vi "UHR-Fleezers Control (host) - Lorentz v5.vi"() -> ()   [LabVIEW 2014] (continued)
                  frame Enabled {
                  }
                }
                n2227 = local read "Actual MCL Inc (V)"() -> (w3371:dbl)
                n2228 = local read "Scan steps (MCL)"() -> (w3376:u64)
                n2229 = Divide "Y Pix/step"(x=w3372, y=w3377) -> (x/y=w3384:dbl)
                n2230 = Divide "Y V/pix"(x=w3371, y=w3384) -> (x/y=w3383:dbl)
                n2231 = Divide "Y half step offset"(x=w3371, y=2.0) -> (x/y=w3385:dbl)
                n2232 = Divide "X pix/step"(x=w3373, y=w3376) -> (x/y=w3382:dbl)
                n2233 = Negate(x=w3385) -> (-x=w3386:dbl)
                n2234 = local read "Initial Y"() -> (w3392:dbl)
                n2235 = Multiply(x=w3374, y=w3383) -> (x*y=w3393:dbl)
                n2236 = Divide "X half step offset"(x=w3371, y=2.0) -> (x/y=w3379:dbl)
                n2237 = Divide "X V/pix"(x=w3371, y=w3382) -> (x/y=w3381:dbl)
                n2238 = Multiply(x=w3371, y=w3376) -> (x*y=w3388:dbl)
                n2239 = Compound Arithmetic op=ADD(w3386, w3393, w3392) -> (w3363:dbl)
                "Pointer Y (V)" <- w3363
                n2240 = Multiply(x=w3381, y=w3375) -> (x*y=w3390:dbl)
                n2241 = Negate(x=w3379) -> (-x=w3378:dbl)
                n2242 = local read "Initial X"() -> (w3391:dbl)
                n2243 = Negate(x=w3390) -> (-x=w3389:dbl)
                n2244 = Compound Arithmetic op=ADD(w3378, w3388, w3391, w3389) -> (w3364:dbl)
                "Pointer X (V)" <- w3364
                n2245 = case shown="True" "Set High F Confocal Spot (X-Y)" {
                  tunnel: w3364 -> [_ w3394]
                  tunnel: w3363 -> [_ w3395]
                  frame False {
                  }
                  frame True {
                    "Confocal Y 2 (V)" <- w3395
                    "Confocal X 2 (V)" <- w3394
                  }
                }
                n2246 = Or(x="Set X Only", y="Set Confocal Spot (X-Y)") -> (x .or. y?=w3367:bool)
                n2247 = Or(x="Set Confocal Spot (X-Y)", y="Set Y Only") -> (x .or. y?=w3366:bool)
                n2248 = case shown="True" w3367 {
                  tunnel: w3364 -> [_ w3396]
                  frame False {
                  }
                  frame True {
                    n2249 = property on="AO2" class="Slide (strict)"("Val(Sgnl)"=w3396) -> ()  [unwired: 2 in, 2 out]
                    "Confocal X 1 (V)" <- w3396
                  }
                }
                n2250 = case shown="True" w3366 {
                  tunnel: w3363 -> [_ w3397]
                  frame False {
                  }
                  frame True {
                    n2251 = property on="AO1" class="Slide (strict)"("Val(Sgnl)"=w3397) -> ()  [unwired: 2 in, 2 out]
                    "Confocal Y 1 (V)" <- w3397
                  }
                }
                n2252 = local write "Set High F Confocal Spot (X-Y)"(w3362) -> ()
                n2253 = local write "Set Confocal Spot (X-Y)"(w3362) -> ()
                n2254 = local write "Set X Only"(w3362) -> ()
                n2255 = local write "Set Y Only"(w3362) -> ()
              }
            }
          }
          frame 3 {
            n2256 = local read "BD 2 Frequency 1 (MHz)"() -> (w3399:dbl)
            n2257 = local read "BD 1 Frequency 1 (MHz)"() -> (w3400:dbl)
            n2258 = local write "Manipulating Trap"(TRUE ("Manipulating Trap")) -> ()
            n2259 = local write "Coords"(T12 {"Horizontal"=0, "Vertical"=0} ("Coords")) -> ()
            n2260 = while {
              tunnel: w3404 -> [w3409]
              tunnel: w3402 -> [w3408]
              tunnel: w3400 -> [w3407]
              tunnel: w3399 -> [w3406]
              tunnel: w3398 -> [w3405]
              stop <- w3410 stop-if-true
              n2261 = event shown="[0] \"Pane\": Mouse Move" {
                selector: _ -> [_ _]
                dyn-events: _ -> [_ _]
                timeout: _ -> [_ _]
                tunnel: ["Force Manip Abort" w3474] -> w3410
                tunnel: w3409 -> [w3417 _]
                tunnel: w3408 -> [w3415 _]
                tunnel: w3407 -> [w3414 _]
                tunnel: w3406 -> [w3413 _]
                tunnel: w3405 -> [w3411 _]
                event Mouse Move {
                  n2262 = event-data() -> ("Time"=w3418:u32, "Coords"=w3419:T12)  [unwired: 3 out]
                  n2263 = Less?(x=w3418, y=w3417) -> (x < y?=w3416:bool)
                  n2264 = case "Makes sure old motion events prior to mouse click aren't used" shown="False" w3416 {
                    tunnel: w3419 -> [w3461 _]
                    tunnel: w3415 -> [w3462 _]
                    tunnel: w3414 -> [w3436 _]
                    tunnel: w3413 -> [w3435 _]
                    tunnel: w3411 -> [w3420 _]
                    frame False {
                      n2265 = Subtract(x=w3461, y=w3462) -> (x-y=w3460:T12)
                      "Coords" <- w3460
                      n2266 = local read "Y RF Frequency Limits (MHz)"() -> (w3421:T23)
                      n2267 = To Double Precision Float(number=w3460) -> (double precision float=w3459:cluster{"Horizontal":dbl, "Vertical":dbl})
                      n2268 = Multiply(x=cluster{"Horizontal":dbl, "Vertical":dbl} {"Horizontal"=-1.0, "Vertical"=1.0}, y="Manipulation Scaling") -> (x*y=w3455:cluster{"Horizontal":dbl, "Vertical":dbl})
                      n2269 = local read "X RF Frequency Limits (MHz)"() -> (w3422:T23)
                      n2270 = Multiply(x=w3459, y=w3455) -> (x*y=w3457:cluster{"Horizontal":dbl, "Vertical":dbl})
                      n2271 = Unbundle By Name(w3457) -> ("Horizontal"=w3452:dbl, "Vertical"=w3456:dbl)
                      n2272 = Unbundle By Name(w3421) -> ("Maximum"=w3424:dbl, "Minimum"=w3423:dbl)
                      n2273 = Boolean To (0,1)(Boolean="Manip. X?") -> (0, 1=w3450:i16)
                      n2274 = Boolean To (0,1)(Boolean="Manip. Y?") -> (0, 1=w3447:i16)
                      n2275 = local read "BD 1 Frequency 2 (MHz)"() -> (w3438:dbl)
                      n2276 = Multiply(x=w3456, y=w3447) -> (x*y=w3449:dbl)
                      n2277 = Multiply(x=w3450, y=w3452) -> (x*y=w3453:dbl)
                      n2278 = local read "BD 2 Frequency 2 (MHz)"() -> (w3437:dbl)
                      n2279 = Unbundle By Name(w3422) -> ("Maximum"=w3426:dbl, "Minimum"=w3425:dbl)
                      n2280 = Add(x=w3435, y=w3449) -> (x+y=w3428:dbl)
                      n2281 = Add(x=w3436, y=w3453) -> (x+y=w3430:dbl)
                      n2282 = In Range and Coerce(upper limit=w3426, x=w3430, lower limit=w3425) -> (coerced(x)=w3429:dbl)  [unwired: 1 out]
                      n2283 = In Range and Coerce(upper limit=w3424, x=w3428, lower limit=w3423) -> (coerced(x)=w3427:dbl)  [unwired: 1 out]
                      n2284 = Subtract(x=w3429, y=w3438) -> (x-y=w3446:dbl)
                      n2285 = Subtract(x=w3427, y=w3437) -> (x-y=w3445:dbl)
                      n2286 = Square(x=w3446) -> (x^2=w3444:dbl)
                      n2287 = Square(x=w3445) -> (x^2=w3443:dbl)
                      n2288 = Add(x=w3444, y=w3443) -> (x+y=w3442:dbl)
                      n2289 = Square Root(x=w3442) -> (sqrt(x)=w3439:dbl)
                      n2290 = In Range and Coerce(upper limit="Limit Max (MHz)", x=w3439, lower limit="Limit Min (MHz)") -> (In Range?=w3432:bool)  [unwired: 1 out]
                      n2291 = Not(x="Limits Enable") -> (.not. x?=w3431:bool)
                      n2292 = Or(x=w3432, y=w3431) -> (x .or. y?=w3433:bool)
                      n2293 = case shown="True" w3433 {
                        tunnel: w3439 -> [_ w3464]
                        tunnel: w3429 -> [_ w3471]
                        tunnel: w3438 -> [_ w3470]
                        tunnel: w3427 -> [_ w3469]
                        tunnel: w3437 -> [_ w3468]
                        tunnel: w3422 -> [_ w3466]
                        tunnel: w3421 -> [_ w3465]
                        tunnel: w3420 -> [_ w3463]
                        frame False {
                        }
                        frame True {
                          n2294 = local read "BD 1 Frequency 3 (MHz)"() -> (w3472:dbl)
                          n2295 = local read "BD 2 Frequency 3 (MHz)"() -> (w3467:dbl)
                          n2296 = local write "Trap Delta (MHz)"(w3464) -> ()
                          n2297 = call "set RF board frequency - interlace.vi"("Board 2 Frequency Limits"=w3465, "Board 1 Frequency Limits"=w3466, "FPGA VI Reference In"=w3463, "Board 2 Frequency 3 (MHz)"=w3467, "Board 1 Frequency 3 (MHz)"=w3472, "Board 2 Frequency 2 (MHz)"=w3468, "Board 2 Frequency 1 (MHz)"=w3469, "Board 1 Frequency 2 (MHz)"=w3470, "Board 1 Frequency 1  (MHz)"=w3471) -> ()  [unwired: 1 in, 2 out]
                          n2298 = local write "BD 2 Frequency 1 (MHz)"(w3469) -> ()
                          n2299 = local write "BD 1 Frequency 1 (MHz)"(w3471) -> ()
                        }
                      }
                    }
                    frame True {
                    }
                  }
                }
                event Mouse Up {
                  n2300 = event-data() -> ("Button"=w3473:u16)  [unwired: 8 out]
                  n2301 = case shown="3" w3473 {
                    tunnel: [FALSE TRUE] -> w3474
                    frame 0, Default {
                    }
                    frame 3 {
                      n2302 = local read "Trap Delta (MHz)"() -> (w3476:dbl)
                      n2303 = property on="Initial delta (MHz)" class="DigNum (strict)"("Val(Sgnl)"=w3476) -> ()  [unwired: 2 in, 2 out]
                      n2304 = local write "Manipulating Trap"(FALSE ("Manipulating Trap")) -> ()
                    }
                  }
                }
              }
            }
          }
        }
      }
      event Timeout {
        n2305 = event-data() -> ()  [unwired: 4 out]
      }
      event "Stop All": Mouse Down {
        n2306 = event-data() -> ()  [unwired: 9 out]
      }
      event Mouse Move {
        n2307 = event-data() -> ()  [unwired: 6 out]
      }
    }
    n2308 = node-c288() -> ()  [unwired: 2 out]
  }
  n2309 = node-c288(3 ("Processor")) -> (w60:T36)  [unwired: 3 out]
  n2310 = node-c288(i64 1 ("Period"), 1 ("Processor")) -> (w68:T36)  [unwired: 2 in, 2 out]
  n2311 = timed-loop "Oscillate Trap/AOM (fishing, conjugate plane alignment)" {
    tunnel: [w3482] -> w65
    timing: w60 -> [_]
    timing-out: [_] -> w59
    tunnel: w21 -> [w3481]
    tunnel: w9 -> [w3480]
    stop <- w3482 stop-if-true
    n2312 = node-c288() -> ()  [unwired: 2 out]
    n2313 = event shown="[2] \"Start assembly line\": Value Change" {
      selector: _ -> [_ _ _ _]
      dyn-events: _ -> [_ _ _ _]
      timeout: _ -> [_ _ _ _]
      tunnel: [FALSE ("Stop All") _ _ w4155] -> w3482
      tunnel: w3481 -> [w3485 _ _ _]
      tunnel: w3480 -> [_ _ w4090 _]
      event "Oscillate Set 1", "Fish for Tether": Value Change {
        n2314 = event-data() -> ()  [unwired: 6 out]
        n2315 = local read "Oscillate Set 1"() -> (w3489:bool)
        n2316 = Or(x=w3489, y="Fish for Tether") -> (x .or. y?=w3487:bool)
        n2317 = case shown="True" w3487 {
          tunnel: "Fish for Tether" -> [_ w3492]
          tunnel: w3485 -> [_ w3490]
          frame False {
          }
          frame True {
            n2318 = case shown="True" w3492 {
              selector: w3492 -> [w3495 w3501]
              tunnel: [w3495 w3501] -> w3491
              frame False {
              }
              frame True {
                n2319 = local write "Scan axis 2"(TRUE) -> ()
                n2320 = local write "Tether"(FALSE ("Tether")) -> ()
                n2321 = local read "Flow ON during cal?"() -> (w3496:bool)
                n2322 = property on="Trap Delta (MHz)" class="DigNum (strict)"("Val(Sgnl)"="Furthest Delta (MHz)") -> ()  [unwired: 2 in, 2 out]
                n2323 = Or(x="Flow ON during \nfishing?", y=w3496) -> (x .or. y?=w3497:bool)
                n2324 = Wait (ms)(milliseconds to wait=u32 500) -> ()  [unwired: 1 out]
                n2325 = property on="Sample Channel\nFlow" class="Bool (strict)"("Val(Sgnl)"=w3497) -> ()  [unwired: 2 in, 2 out]
              }
            }
            n2326 = node-c288() -> (w3494:T36)  [unwired: 1 in, 3 out]
            n2327 = timed-loop "Oscillate AOD" {
              timing: w3494 -> [_]
              timing-out: [_] -> w3493
              tunnel: w3491 -> [w3505]
              tunnel: w3490 -> [w3504]
              i -> [w3513]
              stop <- w3511 stop-if-true
              n2328 = node-c288() -> (w3512:i64)  [unwired: 1 out]
              n2329 = flat-sequence {
                tunnel: w3513 -> [w3540]
                tunnel: w3512 -> [w3539]
                tunnel: w3505 -> [w3523]
                tunnel: [w3523] -> w3510
                tunnel: [w3522] -> w3509
                tunnel: [w3521] -> w3508
                tunnel: [w3518] -> w3506
                tunnel: w3504 -> [w3514]
                tunnel: w3510 -> [w3587]
                tunnel: w3509 -> [w3585]
                tunnel: w3508 -> [w3584]
                tunnel: [w3583] -> w3507
                tunnel: w3506 -> [w3582]
                tunnel: [w3659] -> w3511
                tunnel: w3507 -> [w3658]
                frame #0 {
                  # "w (rad/s)"
                  # "t (s)"
                  n2330 = Divide(x=w3539, y=i64 1000) -> (x/y=w3515:dbl)
                  n2331 = local read "BD 1 Frequency 2 (MHz)"() -> (w3517:dbl)
                  n2332 = Multiply(x="Osc. freq. (Hz)", y=6.283185307179586) -> (x*y=w3537:dbl)
                  n2333 = Multiply(x=w3515, y=w3540) -> (x*y=w3536:dbl)
                  n2334 = Multiply(x=w3537, y=w3536) -> (x*y=w3520:dbl)
                  n2335 = local read "BD 1 Frequency 1 (MHz)"() -> (w3525:dbl)
                  n2336 = case shown="True" w3523 {
                    tunnel: w3520 -> [w3546 w3565]
                    tunnel: w3525 -> [_ w3573]
                    tunnel: w3517 -> [_ w3574]
                    tunnel: [w3543 w3569] -> w3516
                    tunnel: [FALSE w3547] -> w3521
                    tunnel: [0.0 w3561] -> w3518
                    frame False {
                      n2337 = Sine(x=w3546) -> (sin(x)=w3544:dbl)
                      n2338 = Multiply(x=w3544, y="Osc. amp. (MHz)") -> (x*y=w3543:dbl)
                    }
                    frame True {
                      # "trap position goes from 0 to 1 (0 is when it is furthest away, 1 is when closest)\nso we want to test for tether only when farther away, or x < 1"
                      # "quit if taking too long"
                      # "oscillate the trap"
                      # "Test for tether"
                      n2339 = local read "Vec Mean of T1 T2"() -> (w3550:dbl[])
                      "Trigger Signal" <- w3550
                      n2340 = Cosine(x=w3565) -> (cos(x)=w3577:dbl)
                      n2341 = Subtract(x=w3574, y=w3573) -> (x-y=w3572:dbl)
                      n2342 = Decrement(x=w3577) -> (x-1=w3576:dbl)
                      n2343 = Subtract(x=w3572, y="Closest Delta (MHz)") -> (x-y=w3570:dbl)
                      n2344 = Divide(x=w3576, y=-2.0) -> (x/y=w3560:dbl)
                      n2345 = Greater?(x=w3550, y="Stop F (pN)") -> (0:w3567:bool[])
                      n2346 = Multiply(x=w3560, y=w3570) -> (x*y=w3569:dbl)
                      n2347 = Less?(x=w3560, y="Fish mask thresh") -> (x < y?=w3559:bool)
                      n2348 = Boolean To (0,1)(Boolean=w3559) -> (0, 1=w3557:i16)
                      n2349 = Multiply(x=w3557, y=w3550) -> (x*y=w3556:dbl[])
                      n2350 = Divide(x=w3565, y=6.283185307179586) -> (x/y=w3564:dbl)
                      n2351 = Round Toward +Infinity(x=w3564) -> (ceil(x): smallest int >= x=w3561:dbl)
                      "Attempts" <- w3561
                      n2352 = Greater?(x=w3556, y="Stop F (pN) (mask)") -> (0:w3554:bool[])
                      n2353 = Or Array Elements(Boolean array=w3567) -> (logical OR=w3552:bool)
                      n2354 = Or Array Elements(Boolean array=w3554) -> (logical OR=w3551:bool)
                      n2355 = Greater?(x=w3561, y="Attempt Limit") -> (0:w3563:bool)
                      n2356 = case shown="True" w3563 {
                        frame False {
                        }
                        frame True {
                          n2357 = local write "Fish for Tether"(FALSE ("Fish for Tether")) -> ()
                          n2358 = call <vilib>:"Beep.vi"() -> ()  [unwired: 3 in, 9 out]
                          n2359 = local read "Messages"() -> (w3579:string)
                          n2360 = call "Update messages.vi"("Message to add"="Tether fishing timeout." ("Messages"), "Old message string"=w3579) -> ("New message string"=→"Messages":string)
                        }
                      }
                      n2361 = Select(t=w3552, s="Normal (on) or masked test (off)", f=w3551) -> (s? t:f=w3549:bool)
                      n2362 = And(x="Stop Fishing When Tether", y=w3549) -> (x .and. y?=w3547:bool)
                    }
                  }
                  n2363 = local read "BD 2 Frequency 1 (MHz)"() -> (w3524:dbl)
                  n2364 = Select(t=w3525, s="Scan axis 2", f=w3524) -> (s? t:f=w3528:dbl)
                  n2365 = Add(x=w3516, y=w3528) -> (x+y=w3522:dbl)
                  n2366 = Select(t=w3522, s="Scan axis 2", f=w3525) -> (s? t:f=w3531:dbl)
                  n2367 = Select(t=w3524, s="Scan axis 2", f=w3522) -> (s? t:f=w3530:dbl)
                  n2368 = local read "BD 2 Frequency 2 (MHz)"() -> (w3533:dbl)
                  n2369 = local read "BD 2 Frequency 3 (MHz)"() -> (w3532:dbl)
                  n2370 = local read "Y RF Frequency Limits (MHz)"() -> (w3526:T23)
                  n2371 = local read "X RF Frequency Limits (MHz)"() -> (w3527:T23)
                  n2372 = local read "BD 1 Frequency 3 (MHz)"() -> (w3534:dbl)
                  n2373 = call "set RF board frequency - interlace.vi"("Board 2 Frequency Limits"=w3526, "Board 1 Frequency Limits"=w3527, "FPGA VI Reference In"=w3514, "Board 2 Frequency 3 (MHz)"=w3532, "Board 1 Frequency 3 (MHz)"=w3534, "Board 2 Frequency 2 (MHz)"=w3533, "Board 2 Frequency 1 (MHz)"=w3530, "Board 1 Frequency 2 (MHz)"=w3517, "Board 1 Frequency 1  (MHz)"=w3531) -> ()  [unwired: 1 in, 2 out]
                }
                frame #1 {
                  n2374 = And(x=w3587, y=w3584) -> (x .and. y?=w3586:bool)
                  n2375 = case "Only if were fishing and now formed tether" shown="True" w3586 {
                    tunnel: w3585 -> [w3589 w3604]
                    tunnel: [w3588 w3603] -> w3583
                    tunnel: w3582 -> [_ w3599]
                    frame False {
                      n2376 = local read "Fish for Tether"() -> (w3588:bool)
                      n2377 = case shown="False" w3588 {
                        tunnel: w3589 -> [w3590 _]
                        frame False {
                          n2378 = property on="BD 1 Frequency 1 (MHz)" class="DigNum (strict)"("Val(Sgnl)"=w3590) -> ()  [unwired: 2 in, 2 out]
                        }
                        frame True {
                        }
                      }
                    }
                    frame True {
                      w3603 = FALSE ("Fish for Tether")
                      n2379 = call <vilib>:"Beep.vi"() -> ()  [unwired: 3 in, 9 out]
                      n2380 = Number To Decimal String(number=w3599, width (-)=i16 1) -> (decimal integer string=w3597:string)
                      n2381 = Concatenate Strings("Formed tether in ", w3597, " attempt(s)." ("string")) -> (w3594:string)
                      n2382 = local read "Messages"() -> (w3601:string)
                      n2383 = local write "Fish for Tether"(w3603) -> ()
                      n2384 = call "Update messages.vi"("Message to add"=w3594, "Old message string"=w3601) -> ("New message string"=w3600:string)
                      n2385 = local write "Messages"(w3600) -> ()
                      n2386 = Get Date/Time In Seconds() -> (seconds since 1Jan1904=→"Time tether formed":timestamp)
                      n2387 = local read "Flow ON during cal?"() -> (w3591:bool)
                      n2388 = property on="Sample Channel\nFlow" class="Bool (strict)"("Val(Sgnl)"=w3591) -> (error out=w3592:errorcluster)  [unwired: 2 in, 1 out]
                      n2389 = case shown="\"2\", \"3\", \"4\", \"5\", \"6\"" "Then..." {
                        selector: "Then..." -> [_ w3607]
                        tunnel: w3604 -> [w3606 _]
                        tunnel: w3592 -> [_ _]
                        frame "1", Default {
                          n2390 = property on="BD 1 Frequency 1 (MHz)" class="DigNum (strict)"("Val(Sgnl)"=w3606) -> ()  [unwired: 2 in, 2 out]
                        }
                        frame "2", "3", "4", "5", "6" {
                          n2391 = flat-sequence {
                            tunnel: w3607 -> [w3609]
                            frame #0 {
                              n2392 = property on="Trap Delta (MHz)" class="DigNum (strict)"("Val(Sgnl)"="Move to Delta 1 (MHz)") -> ()  [unwired: 2 in, 2 out]
                            }
                            frame #1 {
                              n2393 = case shown="\"5\", \"6\"" w3609 {
                                selector: w3609 -> [w3612 w3622 _]
                                frame "3", "4" {
                                n2394 = flat-sequence {
                                tunnel: w3612 -> [w3613]
                                tunnel: [w3613] -> w3610
                                tunnel: [w3615] -> w3611
                                tunnel: w3610 -> [w3615]
                                tunnel: w3611 -> [w3619]
                                frame #0 {
                                n2395 = property on="Green Laser ON" class="Bool (strict)"("Val(Sgnl)"=TRUE ("Value (Signaling)")) -> ()  [unwired: 2 in, 2 out]
                                }
                                frame #1 {
                                n2396 = Multiply(x="Wait Before Save (s)", y=u32 1000 ("x")) -> (x*y=w3617:u32)
                                n2397 = Wait (ms)(milliseconds to wait=w3617) -> ()  [unwired: 1 out]
                                }
                                frame #2 {
                                n2398 = property on="Start Saving" class="Bool (strict)"("Value"=TRUE ("Start Saving")) -> ()  [unwired: 2 in, 2 out]
                                n2399 = case shown="\"4\"" w3619 {
                                frame Default {
                                }
                                frame "4" {
                                n2400 = property on="Fl. Triggered..." class="Bool (strict)"("Val(Sgnl)"=TRUE ("Value (Signaling)")) -> ()  [unwired: 2 in, 2 out]
                                }
                                }
                                }
                                }
                                }
                                frame "5", "6" {
                                n2401 = stacked-sequence {
                                tunnel: w3622 -> [_ _ _ _ _ _ w3634]
                                frame #0 {
                                n2402 = Replace Array Subset(array=u32[] [0] ("Index Values"), new element="Raster Set Upon Tether", index=0) -> (w3623:u32[])
                                n2403 = property on="Saved AOD Raster Scan Parameter Sets" class="Arr (strict)"("Index Values"=w3623) -> ()  [unwired: 2 in, 2 out]
                                }
                                frame #1 {
                                n2404 = Wait (ms)(milliseconds to wait=u32 500) -> ()  [unwired: 1 out]
                                }
                                frame #2 {
                                n2405 = property on="Load parameters" class="Bool (strict)"("Val(Sgnl)"=TRUE ("Value (Signaling)")) -> ()  [unwired: 2 in, 2 out]
                                n2406 = case shown="True" "Green ON During Raster" {
                                frame False {
                                }
                                frame True {
                                n2407 = property on="Green Laser ON" class="Bool (strict)"("Val(Sgnl)"=TRUE ("Value (Signaling)")) -> ()  [unwired: 2 in, 2 out]
                                }
                                }
                                }
                                frame #3 {
                                n2408 = Wait (ms)(milliseconds to wait=u32 500) -> ()  [unwired: 1 out]
                                }
                                frame #4 {
                                n2409 = property on="Trap Raster Scan" class="Bool (strict)"("Val(Sgnl)"=TRUE ("Value (Signaling)")) -> ()  [unwired: 2 in, 2 out]
                                }
                                frame #5 {
                                n2410 = Wait (ms)(milliseconds to wait=u32 2000) -> ()  [unwired: 1 out]
                                }
                                frame #6 {
                                n2411 = flat-sequence {
                                tunnel: w3634 -> [w3641]
                                frame #0 {
                                n2412 = while {
                                stop <- w3637 stop-if-true
                                n2413 = local read "Raster Scanning..."() -> (w3636:bool)
                                n2414 = local read "Saving..."() -> (w3639:bool)
                                n2415 = Wait (ms)(milliseconds to wait=u32 100) -> ()  [unwired: 1 out]
                                n2416 = Not(x=w3639) -> (.not. x?=w3638:bool)
                                n2417 = Not(x=w3636) -> (.not. x?=w3635:bool)
                                n2418 = And(x=w3638, y=w3635) -> (x .and. y?=w3637:bool)
                                }
                                }
                                frame #1 {
                                n2419 = local read "Tether"() -> (w3642:bool)
                                n2420 = case shown="True" w3642 {
                                tunnel: w3641 -> [_ w3644]
                                frame False {
                                n2421 = property on="Fish for Tether" class="Bool (strict)"("Val(Sgnl)"="Fish again after \nraster break?") -> ()  [unwired: 2 in, 2 out]
                                }
                                frame True {
                                n2422 = stacked-sequence {
                                tunnel: w3644 -> [_ w3648 _ _]
                                frame #0 {
                                n2423 = property on="Trap Delta (MHz)" class="DigNum (strict)"("Val(Sgnl)"="Move to Delta 2 (MHz)") -> ()  [unwired: 2 in, 2 out]
                                n2424 = case shown="True" "Flow ON after\ntether testing?" {
                                frame False {
                                }
                                frame True {
                                n2425 = property on="Sample Channel\nFlow" class="Bool (strict)"("Val(Sgnl)"=TRUE ("Value (Signaling)")) -> ()  [unwired: 2 in, 2 out]
                                }
                                }
                                }
                                frame #1 {
                                n2426 = flat-sequence {
                                tunnel: w3648 -> [w3650]
                                frame #0 {
                                n2427 = Wait (ms)(milliseconds to wait=u32 500) -> ()  [unwired: 1 out]
                                }
                                frame #1 {
                                n2428 = case shown="\"6\"" w3650 {
                                frame Default {
                                }
                                frame "6" {
                                n2429 = property on="Green Laser ON" class="Bool (strict)"("Val(Sgnl)"=TRUE ("Green Laser ON/Interlacing")) -> ()  [unwired: 2 in, 2 out]
                                }
                                }
                                }
                                frame #2 {
                                n2430 = Wait (ms)(milliseconds to wait=u32 500) -> ()  [unwired: 1 out]
                                }
                                frame #3 {
                                n2431 = local write "Start Saving"("Save at end (5, 6)") -> ()
                                }
                                }
                                }
                                frame #2 {
                                n2432 = local read "Bead Sep. Int. Time (s)"() -> (w3656:dbl)
                                n2433 = Multiply(x=w3656, y=1000.0) -> (x*y=w3655:dbl)
                                n2434 = Wait (ms)(milliseconds to wait=w3655) -> ()  [unwired: 1 out]
                                }
                                frame #3 {
                                n2435 = property on="Remove Offset" class="Bool (strict)"("Val(Sgnl)"=TRUE ("Value (Signaling)")) -> ()  [unwired: 2 in, 2 out]
                                }
                                }
                                }
                                }
                                }
                                }
                                }
                                }
                                }
                                frame "2", Default {
                                }
                              }
                            }
                          }
                        }
                      }
                      "Tether" <- "Tether Alarm?"
                    }
                  }
                }
                frame #2 {
                  n2436 = local read "Oscillate Set 1"() -> (w3663:bool)
                  n2437 = local read "Stop All"() -> (w3661:bool)
                  n2438 = Or(x=w3663, y=w3658) -> (x .or. y?=w3660:bool)
                  n2439 = Not(x=w3660) -> (.not. x?=w3662:bool)
                  n2440 = Compound Arithmetic op=OR(w3661, w3662) -> (w3659:bool)
                }
              }
              n2441 = node-c288() -> ()  [unwired: 2 out]
            }
            n2442 = node-c288(w3493) -> ()  [unwired: 1 out]
          }
        }
      }
      event "Fl. Triggered...": Value Change {
        n2443 = event-data() -> ()  [unwired: 7 out]
        n2444 = case shown="True" "Fl. Triggered..." {
          frame False {
          }
          frame True {
            n2445 = node-c288() -> (w3674:T36)  [unwired: 4 out]
            n2446 = timed-loop {
              timing: w3674 -> [_]
              timing-out: [_] -> w3673
              tunnel: "Action" -> [w3682]
              shift-right: [w3679] -> _
              shift-left: u8 255 -> [w3681]
              shift-right: [w3676] -> _
              shift-left: 255 -> [w3678]
              stop <- w3675 stop-if-true
              # "Reset confocal spot"
              n2447 = node-c288() -> ()  [unwired: 2 out]
              n2448 = flat-sequence {
                tunnel: w3682 -> [w3702]
                tunnel: w3681 -> [w3701]
                tunnel: [w3700] -> w3680
                tunnel: w3678 -> [w3687]
                tunnel: [w3686] -> w3677
                tunnel: [w4081] -> w3675
                tunnel: w3680 -> [w4080]
                tunnel: [w4080] -> w3679
                tunnel: [w4079] -> w3676
                tunnel: w3677 -> [w4079]
                frame #0 {
                  n2449 = local read "Delta Fl. 2"() -> (w3699:dbl)
                  n2450 = local read "Delta Fl. 1"() -> (w3694:dbl)
                  n2451 = Multiply(x="Fl. Delta Thresh. (kHz)", y=1000.0) -> (x*y=w3689:dbl)
                  n2452 = Select(t=w3694, s="APD to Watch", f=w3699) -> (s? t:f=w3690:dbl)
                  n2453 = Greater?(x=w3690, y=w3689) -> (0:w3695:bool)
                  n2454 = Or(x="Force Yank", y=w3695) -> (x .or. y?=w3693:bool)
                  n2455 = And(x=w3693, y="Yank when?") -> (x .and. y?=w3691:bool)
                  n2456 = case shown="True" w3691 {
                    tunnel: w3702 -> [w3705 w3906]
                    tunnel: w3701 -> [w3707 w3902]
                    tunnel: [w3707 w3900] -> w3700
                    tunnel: w3690 -> [w3713 _]
                    tunnel: w3689 -> [w3712 _]
                    tunnel: "Force Yank" -> [w3710 _]
                    tunnel: w3687 -> [w3709 w3899]
                    tunnel: [w3708 w3899] -> w3686
                    frame False {
                      n2457 = Negate(x=w3712) -> (-x=w3704:dbl)
                      n2458 = local write "Fl. High"(TRUE ("Fl. High")) -> ()
                      n2459 = Less?(x=w3713, y=w3704) -> (x < y?=w3711:bool)
                      n2460 = Or(x=w3710, y=w3711) -> (x .or. y?=w3706:bool)
                      n2461 = case shown="True" w3706 {
                        tunnel: w3709 -> [w3714 w3724]
                        tunnel: [w3714 w3723] -> w3708
                        tunnel: w3705 -> [_ w3722]
                        frame False {
                        }
                        frame True {
                          n2462 = flat-sequence {
                            tunnel: w3724 -> [w3730]
                            tunnel: w3722 -> [w3727]
                            tunnel: [w3729] -> w3721
                            tunnel: [w3728] -> w3720
                            tunnel: [w3727] -> w3719
                            tunnel: w3718 -> [w3726]
                            tunnel: [w3726] -> w3717
                            tunnel: w3716 -> [w3725]
                            tunnel: [w3725] -> w3715
                            tunnel: [w3801] -> w3723
                            tunnel: w3721 -> [w3801]
                            tunnel: w3720 -> [w3800]
                            tunnel: w3719 -> [w3799]
                            tunnel: w3717 -> [w3798]
                            tunnel: w3715 -> [w3797]
                            frame #0 {
                              n2463 = call <vilib>:"Beep.vi"() -> ()  [unwired: 12 in]
                              n2464 = local write "Waiting"(FALSE ("Waiting")) -> ()
                              n2465 = Increment(x=w3730) -> (x+1=w3729:i32)
                              n2466 = case shown="\"Image\"" w3727 {
                                tunnel: w3729 -> [_ w3735 _]
                                frame "Alarm", Default {
                                }
                                frame "Yank" {
                                n2467 = flat-sequence {
                                tunnel: w3735 -> [w3738]
                                tunnel: [w3737] -> w3734
                                tunnel: [w3736] -> w3733
                                tunnel: w3734 -> [w3748]
                                tunnel: w3733 -> [w3749]
                                frame #0 {
                                n2468 = local read "Yank Delay (s)"() -> (w3741:dbl)
                                n2469 = local read "N Array El"() -> (w3736:u8)
                                n2470 = Quotient & Remainder(x=w3738, y=w3736) -> (x-y*floor(x/y)=w3737:i32)  [unwired: 1 out]
                                n2471 = Multiply(x=w3741, y=1000.0) -> (x*y=w3739:dbl)
                                n2472 = Wait (ms)(milliseconds to wait=w3739) -> ()  [unwired: 1 out]
                                }
                                frame #1 {
                                n2473 = local read "Yank to which?"() -> (w3743:bool)
                                n2474 = local read "Random Choice"() -> (w3753:bool)
                                n2475 = local read "Yank to Trap Delta (MHz)"() -> (w3746:dbl[])
                                n2476 = local read "Yank to SP"() -> (w3747:dbl[])
                                n2477 = Random Number (0-1)() -> (number: 0 to 1=w3752:dbl)
                                n2478 = Multiply(x=w3749, y=w3752) -> (x*y=w3751:dbl)
                                n2479 = Round Toward -Infinity(1:w3751) -> (0:w3750:dbl)
                                n2480 = Select(t=w3750, s=w3753, f=w3748) -> (s? t:f=w3744:dbl)
                                n2481 = Select(t=w3746, s=w3743, f=w3747) -> (s? t:f=w3745:dbl[])
                                n2482 = Index Array(array=w3745, index=w3744) -> (element=w3742:dbl)
                                n2483 = case shown="True" w3743 {
                                tunnel: w3742 -> [w3754 w3781]
                                frame False {
                                n2484 = flat-sequence {
                                tunnel: w3754 -> [w3755]
                                frame #0 {
                                n2485 = property on="Trap Pos FB SP" class="DigNum (strict)"("Val(Sgnl)"=w3755) -> ()  [unwired: 2 in, 2 out]
                                }
                                frame #1 {
                                n2486 = Wait (ms)(milliseconds to wait=u32 700) -> ()  [unwired: 1 out]
                                }
                                frame #2 {
                                n2487 = local read "Action (%)"() -> (w3760:dbl)
                                n2488 = Absolute Value(x=w3760) -> (abs(x)=w3759:dbl)
                                n2489 = Greater?(x=w3759, y=70.0) -> (0:w3757:bool)
                                n2490 = property on="Remove Action Offset" class="Bool (strict)"("Val(Sgnl)"=w3757) -> ()  [unwired: 2 in, 2 out]
                                }
                                frame #3 {
                                n2491 = for {
                                N: 4 -> [_]
                                n2492 = flat-sequence {
                                frame #0 {
                                n2493 = Wait (ms)(milliseconds to wait=u32 500) -> ()  [unwired: 1 out]
                                }
                                frame #1 {
                                n2494 = local read "Action (%)"() -> (w3766:dbl)
                                n2495 = Absolute Value(x=w3766) -> (abs(x)=w3765:dbl)
                                n2496 = Greater?(x=w3765, y=70.0) -> (0:w3763:bool)
                                n2497 = property on="Remove Action Offset" class="Bool (strict)"("Val(Sgnl)"=w3763) -> ()  [unwired: 2 in, 2 out]
                                }
                                }
                                }
                                }
                                frame #4 {
                                n2498 = Wait (ms)(milliseconds to wait=u32 500) -> ()  [unwired: 1 out]
                                }
                                frame #5 {
                                n2499 = local read "Mean"() -> (w3774:dbl)
                                n2500 = Greater?(x=w3774, y=11.0) -> (0:w3768:bool)
                                n2501 = Not(x=w3768) -> (.not. x?=w3769:bool)
                                n2502 = And(x=w3769, y="Shift confocal") -> (x .and. y?=w3771:bool)
                                n2503 = And(x=w3768, y="Shift confocal") -> (x .and. y?=w3772:bool)
                                n2504 = case shown="True" w3772 {
                                frame False {
                                }
                                frame True {
                                n2505 = local read "Confocal Y 2 (V)"() -> (w3778:dbl)
                                n2506 = local read "Confocal X 2 (V)"() -> (w3777:dbl)
                                n2507 = property on="AO1" class="Slide (strict)"("Val(Sgnl)"=w3778) -> ()  [unwired: 2 in, 2 out]
                                n2508 = property on="AO2" class="Slide (strict)"("Val(Sgnl)"=w3777) -> ()  [unwired: 2 in, 2 out]
                                }
                                }
                                n2509 = case shown="True" w3771 {
                                frame False {
                                }
                                frame True {
                                n2510 = local read "Confocal Y 1 (V)"() -> (w3776:dbl)
                                n2511 = local read "Confocal X 1 (V)"() -> (w3775:dbl)
                                n2512 = property on="AO1" class="Slide (strict)"("Val(Sgnl)"=w3776) -> ()  [unwired: 2 in, 2 out]
                                n2513 = property on="AO2" class="Slide (strict)"("Val(Sgnl)"=w3775) -> ()  [unwired: 2 in, 2 out]
                                }
                                }
                                }
                                frame #6 {
                                n2514 = Wait (ms)(milliseconds to wait=u32 1500) -> ()  [unwired: 1 out]
                                }
                                frame #7 {
                                n2515 = property on="Rem fb disp offset" class="Bool (strict)"("Val(Sgnl)"=TRUE ("Value (Signaling)")) -> ()  [unwired: 2 in, 2 out]
                                }
                                }
                                }
                                frame True {
                                n2516 = flat-sequence {
                                tunnel: w3781 -> [w3782]
                                frame #0 {
                                n2517 = property on="Trap Delta (MHz)" class="DigNum (strict)"("Val(Sgnl)"=w3782) -> ()  [unwired: 2 in, 2 out]
                                }
                                frame #1 {
                                n2518 = Wait (ms)(milliseconds to wait=u32 500) -> ()  [unwired: 1 out]
                                }
                                frame #2 {
                                n2519 = local read "Shift confocal"() -> (w3788:bool)
                                n2520 = local read "Mean"() -> (w3790:dbl)
                                n2521 = Greater?(x=w3790, y=11.0) -> (0:w3787:bool)
                                n2522 = Not(x=w3787) -> (.not. x?=w3786:bool)
                                n2523 = And(x=w3786, y=w3788) -> (x .and. y?=w3784:bool)
                                n2524 = And(x=w3787, y=w3788) -> (x .and. y?=w3785:bool)
                                n2525 = case shown="True" w3785 {
                                frame False {
                                }
                                frame True {
                                n2526 = local read "Confocal Y 2 (V)"() -> (w3794:dbl)
                                n2527 = local read "Confocal X 2 (V)"() -> (w3793:dbl)
                                n2528 = property on="AO2" class="Slide (strict)"("Val(Sgnl)"=w3793) -> ()  [unwired: 2 in, 2 out]
                                n2529 = property on="AO1" class="Slide (strict)"("Val(Sgnl)"=w3794) -> ()  [unwired: 2 in, 2 out]
                                }
                                }
                                n2530 = case shown="True" w3784 {
                                frame False {
                                }
                                frame True {
                                n2531 = local read "Confocal X 1 (V)"() -> (w3791:dbl)
                                n2532 = local read "Confocal Y 1 (V)"() -> (w3792:dbl)
                                n2533 = property on="AO2" class="Slide (strict)"("Val(Sgnl)"=w3791) -> ()  [unwired: 2 in, 2 out]
                                n2534 = property on="AO1" class="Slide (strict)"("Val(Sgnl)"=w3792) -> ()  [unwired: 2 in, 2 out]
                                }
                                }
                                }
                                }
                                }
                                }
                                }
                                }
                                }
                                frame "Image" {
                                n2535 = property on="Confocal Image" class="Bool (strict)"("Val(Sgnl)"=TRUE ("Value (Signaling)")) -> ()  [unwired: 2 in, 2 out]
                                }
                              }
                              n2536 = local write "Fl. High"(FALSE ("Fl. High")) -> ()
                              n2537 = local read "Time (s)"() -> (w3728:dbl)
                            }
                            frame #1 {
                              n2538 = case shown="True" "Auto F Reset" {
                                tunnel: w3800 -> [_ w3805]
                                tunnel: w3799 -> [_ w3804]
                                tunnel: w3798 -> [_ w3803]
                                tunnel: w3797 -> [_ w3802]
                                frame False {
                                }
                                frame True {
                                n2539 = node-c288() -> (w3807:T36)  [unwired: 4 in]
                                n2540 = timed-loop {
                                timing: w3807 -> [_]
                                timing-out: [_] -> w3806
                                tunnel: w3805 -> [w3812]
                                tunnel: w3804 -> [w3811]
                                tunnel: w3803 -> [w3810]
                                tunnel: w3802 -> [w3809]
                                stop <- w3808 stop-if-true
                                n2541 = node-c288() -> ()  [unwired: 1 in, 1 out]
                                n2542 = local read "Fl. Delta Thresh. (kHz)"() -> (w3821:dbl)
                                n2543 = local read "APD to Watch"() -> (w3822:bool)
                                n2544 = local read "Delta Fl. 1"() -> (w3823:dbl)
                                n2545 = local read "Delta Fl. 2"() -> (w3824:dbl)
                                n2546 = local read "Fl. Triggered..."() -> (w3815:bool)
                                n2547 = local read "Stop All"() -> (w3816:bool)
                                n2548 = local read "Reset Force"() -> (w3814:bool)
                                n2549 = Multiply(x=w3821, y=1000.0) -> (x*y=w3819:dbl)
                                n2550 = Select(t=w3823, s=w3822, f=w3824) -> (s? t:f=w3818:dbl)
                                n2551 = Not(x=w3815) -> (.not. x?=w3813:bool)
                                n2552 = Greater?(x=w3818, y=w3819) -> (0:w3817:bool)
                                n2553 = Compound Arithmetic op=OR(w3817, w3816, w3813, w3814) -> (w3808:bool)
                                n2554 = case shown="True" w3808 {
                                tunnel: w3812 -> [_ w3828]
                                tunnel: w3811 -> [_ w3832]
                                tunnel: w3810 -> [_ w3831]
                                tunnel: w3809 -> [_ w3830]
                                frame False {
                                }
                                frame True {
                                n2555 = case shown="\"Yank\"" w3832 {
                                tunnel: w3831 -> [_ w3842]
                                tunnel: w3830 -> [_ w3840]
                                frame "Image", Default {
                                }
                                frame "Yank" {
                                n2556 = flat-sequence {
                                tunnel: [w3845] -> w3843
                                tunnel: w3842 -> [w3845]
                                tunnel: [w3844] -> w3841
                                tunnel: w3840 -> [w3844]
                                tunnel: w3843 -> [w3851]
                                tunnel: w3841 -> [w3849]
                                frame #0 {
                                n2557 = local read "Yank Delay (s)"() -> (w3848:dbl)
                                n2558 = Multiply(x=w3848, y=1000.0) -> (x*y=w3846:dbl)
                                n2559 = Wait (ms)(milliseconds to wait=w3846) -> ()  [unwired: 1 out]
                                }
                                frame #1 {
                                n2560 = local read "Yank to which?"() -> (w3850:bool)
                                n2561 = case shown="False" w3850 {
                                tunnel: w3851 -> [_ w3879]
                                tunnel: w3849 -> [w3852 _]
                                frame False {
                                n2562 = flat-sequence {
                                tunnel: w3852 -> [w3853]
                                frame #0 {
                                n2563 = property on="Trap Pos FB SP" class="DigNum (strict)"("Val(Sgnl)"=w3853) -> ()  [unwired: 2 in, 2 out]
                                }
                                frame #1 {
                                n2564 = Wait (ms)(milliseconds to wait=u32 700) -> ()  [unwired: 1 out]
                                }
                                frame #2 {
                                n2565 = local read "Action (%)"() -> (w3858:dbl)
                                n2566 = Absolute Value(x=w3858) -> (abs(x)=w3857:dbl)
                                n2567 = Greater?(x=w3857, y=70.0) -> (0:w3855:bool)
                                n2568 = property on="Remove Action Offset" class="Bool (strict)"("Val(Sgnl)"=w3855) -> ()  [unwired: 2 in, 2 out]
                                }
                                frame #3 {
                                n2569 = for {
                                N: 4 -> [_]
                                n2570 = flat-sequence {
                                frame #0 {
                                n2571 = Wait (ms)(milliseconds to wait=u32 500) -> ()  [unwired: 1 out]
                                }
                                frame #1 {
                                n2572 = local read "Action (%)"() -> (w3864:dbl)
                                n2573 = Absolute Value(x=w3864) -> (abs(x)=w3863:dbl)
                                n2574 = Greater?(x=w3863, y=70.0) -> (0:w3861:bool)
                                n2575 = property on="Remove Action Offset" class="Bool (strict)"("Val(Sgnl)"=w3861) -> ()  [unwired: 2 in, 2 out]
                                }
                                }
                                }
                                }
                                frame #4 {
                                n2576 = Wait (ms)(milliseconds to wait=u32 500) -> ()  [unwired: 1 out]
                                }
                                frame #5 {
                                n2577 = local read "Shift confocal"() -> (w3869:bool)
                                n2578 = local read "Mean"() -> (w3872:dbl)
                                n2579 = Greater?(x=w3872, y=11.0) -> (0:w3868:bool)
                                n2580 = Not(x=w3868) -> (.not. x?=w3867:bool)
                                n2581 = And(x=w3868, y=w3869) -> (x .and. y?=w3870:bool)
                                n2582 = And(x=w3867, y=w3869) -> (x .and. y?=w3866:bool)
                                n2583 = case shown="True" w3870 {
                                frame False {
                                }
                                frame True {
                                n2584 = local read "Confocal X 2 (V)"() -> (w3875:dbl)
                                n2585 = local read "Confocal Y 2 (V)"() -> (w3876:dbl)
                                n2586 = property on="AO2" class="Slide (strict)"("Val(Sgnl)"=w3875) -> ()  [unwired: 2 in, 2 out]
                                n2587 = property on="AO1" class="Slide (strict)"("Val(Sgnl)"=w3876) -> ()  [unwired: 2 in, 2 out]
                                }
                                }
                                n2588 = case shown="True" w3866 {
                                frame False {
                                }
                                frame True {
                                n2589 = local read "Confocal Y 1 (V)"() -> (w3874:dbl)
                                n2590 = local read "Confocal X 1 (V)"() -> (w3873:dbl)
                                n2591 = property on="AO1" class="Slide (strict)"("Val(Sgnl)"=w3874) -> ()  [unwired: 2 in, 2 out]
                                n2592 = property on="AO2" class="Slide (strict)"("Val(Sgnl)"=w3873) -> ()  [unwired: 2 in, 2 out]
                                }
                                }
                                }
                                frame #6 {
                                n2593 = Wait (ms)(milliseconds to wait=u32 1500) -> ()  [unwired: 1 out]
                                }
                                frame #7 {
                                n2594 = property on="Rem fb disp offset" class="Bool (strict)"("Val(Sgnl)"=TRUE ("Value (Signaling)")) -> ()  [unwired: 2 in, 2 out]
                                }
                                }
                                }
                                frame True {
                                n2595 = flat-sequence {
                                tunnel: w3879 -> [w3880]
